vi "select UDP port.vi"(9 "force UDP port":bool, 10 "receiver port (if not in target or forced, use global default)":u16, 11 "message":T1) -> (3 "receiver port (global default)":u16)   [LabVIEW 2013, in "AMC.lvlib"]
uses:
  AMC.lvlib
  Message.ctl
  <vilib>/NI/Tools/Keyed Array/KeyedArray.ctl
  Globals.vi
  <vilib>/NI/Tools/Keyed Array/Tools_KeyedArray.lvlib
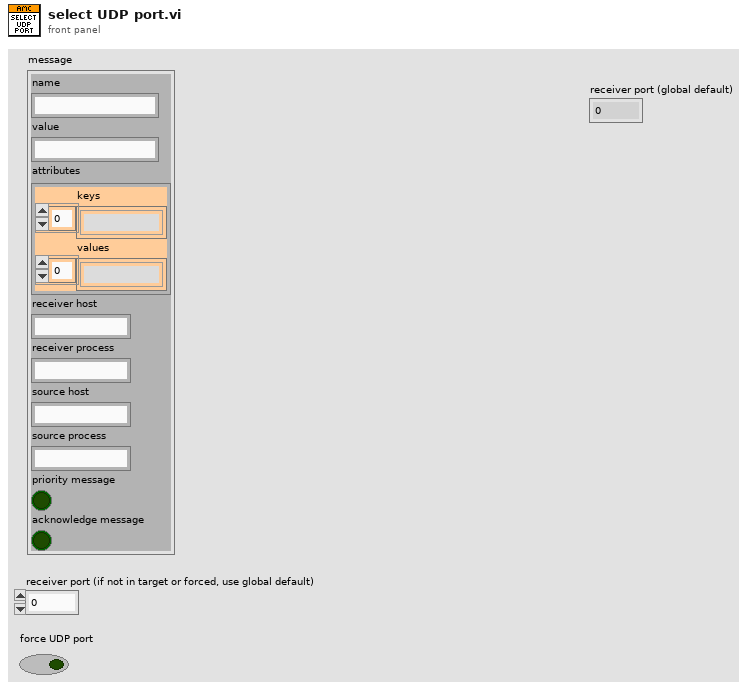
[diagram p1: front panel]
types:
  T1 = typedef "AMC.lvlib/Message.ctl" = cluster{"name":string, "value":string, "attributes":T2, "receiver host":string, "receiver process":string, "source host":string, "source process":string, "priority message":bool, "acknowledge message":bool}
  T2 = typedef "Tools_KeyedArray.lvlib/KeyedArray.ctl" = cluster{"keys":string[], "values":string[]}
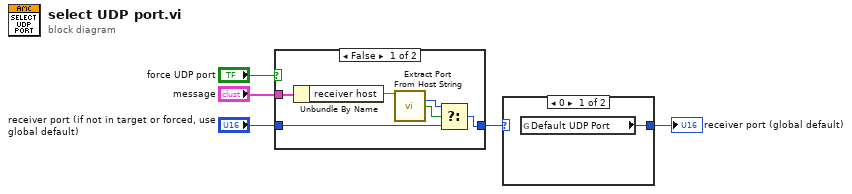
[diagram p0: block diagram]
diagram:
  n1 = case shown="False" "force UDP port" {
    tunnel: [w6 w12] -> w3
    tunnel: "receiver port (if not in target or forced, use global default)" -> [w7 w12]
    tunnel: "message" -> [w11 _]
    frame False {
      n2 = Unbundle By Name(w11) -> ("receiver host"=w10:string)
      n3 = call "Extract Port From Host String.vi"("host in"=w10) -> ("port"=w8:u16, "found?"=w9:bool)  [unwired: 12 in, 1 out]
      n4 = Select(t=w8, s=w9, f=w7) -> (s? t:f=w6:u16)
    }
    frame True {
    }
  }
  n5 = case shown="0" w3 {
    selector: w3 -> [_ w14]
    tunnel: [w13 w14] -> w5
    frame 0 {
      n6 = global read "Globals.vi" "Default UDP Port"() -> (w13:u16)
    }
    frame Default {
    }
  }
  "receiver port (global default)" <- w5
